vi "Find window with lowest SD.vi"(11 "Input Data":dynamicdata(waveform)) -> (2 "Index of min SD":i32, 3 "Minimum SD":dbl)   [LabVIEW 2016]
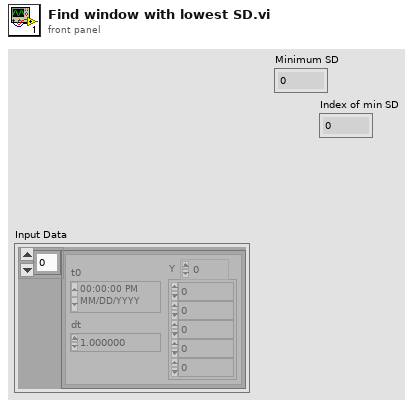
[diagram p1: front panel]
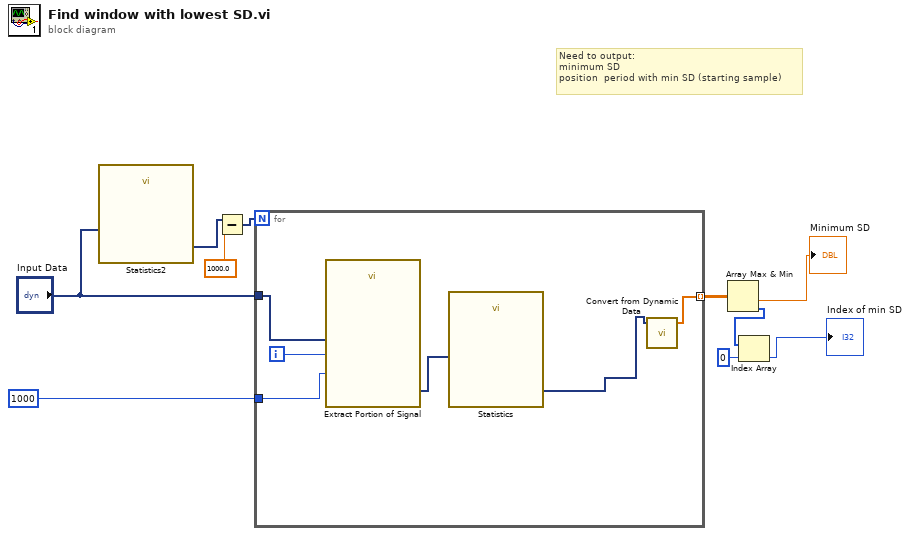
[diagram p0: block diagram]
diagram:
  # "Need to output:\nminimum SD\nposition  period with min SD (starting sample)"
  n1 = call "Statistics2"("Signals"="Input Data") -> ("Total Samples"=w5:dynamicdata)  [unwired: 25 in, 1 out]
  n2 = Subtract(x=w5, y=1000.0) -> (x-y=w6:dynamicdata)
  n3 = for {
    N: w6 -> [_]
    tunnel: "Input Data" -> [w16]
    tunnel: 1000 ("#samples for SW period") -> [w15]
    tunnel: [w11] -> w9 mode=indexing
    i -> [w13]
    n4 = call "Extract Portion of Signal"("Samples"=w15, "Begin Sample"=w13, "Signals"=w16) -> ("Section"=w14:dynamicdata)  [unwired: 7 in, 1 out]
    n5 = call "Statistics"("Signals"=w14) -> ("Standard Dev"=w12:dynamicdata)  [unwired: 24 in, 2 out]
    n6 = call "Convert from Dynamic Data"("Dynamic Data Type"=w12) -> ("Array"=w11:dbl[])  [unwired: 3 out]
  }
  n7 = Array Max & Min(array=w9) -> (min value=→"Minimum SD":dbl, min index (indices)=w3:i32[])  [unwired: 2 out]
  n8 = Index Array(array=w3, index=0) -> (element=→"Index of min SD":i32)
